vi "Archive Graduated Student.vi"(11 "BYU ID # In":string) -> ()   [LabVIEW 2019]
uses:
  Controls/Table Data Types/User Data Type.ctl
  Controls/Table Data Types/User Archive Data Type.ctl
  <vilib>/addons/database/Connection.llb/DB Tools Open Connec (String).vi
  <vilib>/addons/database/_DB Variant To Data/Database Variant To Data.xnode
  <vilib>/addons/database/NI_Database_API.lvlib
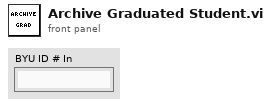
[diagram p1: front panel]
types:
  T1 = typedef "User Archive Data Type.ctl" = cluster{"BYU ID #":string, "First Name":string, "Last Name":string, "Phone Number":string, "Email":string, "Department":string, "Graduation Status":string, "Anticipated Graduation Year":string, "Credit Score":dbl, "Date Added":string, "Graduation Clearance Date":string, "Picture File Name":string, "Date Archived":string}
  T2 = typedef "User Data Type.ctl" = cluster{"BYU ID #":string, "First Name":string, "Last Name":string, "Phone Number":string, "Email":string, "Department":string, "Graduation Status":string, "Anticipated Graduation Year":string, "Credit Score":dbl, "Date Added":string, "Graduation Clearance Date":string, "Picture File Name":string, "User Comments":string}
  T3 = typedef "NI_Database_API.lvlib/Conn ObjectReference.ctl" = refnum<k1>
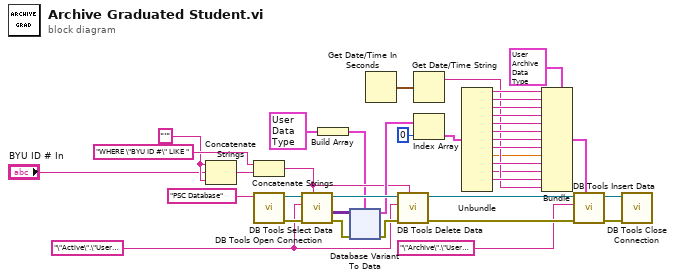
[diagram p0: block diagram]
diagram:
  w2 = "'" ("string")
  w16 = "\"Active\".\"Users\""
  n1 = Concatenate Strings(w2, "BYU ID # In", w2) -> (w3:string)
  n2 = Concatenate Strings("WHERE \"BYU ID #\" LIKE " ("string"), w3) -> (w17:string)
  n3 = call-poly <vilib>:"DB Tools Open Connection.vi"("connection information"="PSC Database") -> ("error out"=w37:errorcluster, "connection reference"=w38:T3)  [unwired: 7 in]
  n4 = call <vilib>:"DB Tools Select Data.vi"("condition"=w17, "error in (no error)"=w37, "table"=w16, "connection reference"=w38) -> ("error out"=w34:errorcluster, "data"=w35:variant[][], "connection reference out"=w36:T3)  [unwired: 2 in]
  n5 = Build Array(T2 {"BYU ID #"="", "First Name"="", "Last Name"="", "Phone Number"="", "Email"="", "Department"="", "Graduation Status"="", "Anticipated Graduation Year"="", "Credit Score"=0.0, "Date Added"="", "Graduation Clearance Date"="", "Picture File Name"="", "User Comments"=""} ("Array")) -> (w8:T2[])
  n6 = xnode "Database Variant To Data"("database variant"=w35, "error in (no error)"=w34, "type"=w8) -> ("data"=w32:T2[], "error out"=w33:errorcluster)
  n7 = Get Date/Time In Seconds() -> (seconds since 1Jan1904=w19:timestamp)
  n8 = call <vilib>:"DB Tools Delete Data.vi"("condition"=w17, "error in (no error)"=w33, "table"=w16, "connection reference"=w36) -> ("error out"=w13:errorcluster, "connection reference out"=w14:T3)  [unwired: 6 in]
  n9 = Get Date/Time String(seconds (now)=w19) -> (date string=w18:string)  [unwired: 2 in, 1 out]
  n10 = Index Array(array=w32, index=0) -> (element=w30:T2)
  n11 = Unbundle(w30) -> ("BYU ID #"=w29:string, "First Name"=w28:string, "Last Name"=w27:string, "Phone Number"=w26:string, "Email"=w25:string, "Department"=w24:string, "Graduation Status"=w23:string, "Anticipated Graduation Year"=w22:string, "Credit Score"=w6:dbl, "Date Added"=w21:string, "Graduation Clearance Date"=w5:string, "Picture File Name"=w20:string)  [unwired: 1 out]
  n12 = Bundle(cluster=T1 {"BYU ID #"="", "First Name"="", "Last Name"="", "Phone Number"="", "Email"="", "Department"="", "Graduation Status"="", "Anticipated Graduation Year"="", "Credit Score"=0.0, "Date Added"="", "Graduation Clearance Date"="", "Picture File Name"="", "Date Archived"=""} ("USER ARCHIVE DATA TYPE"), "BYU ID #"=w29, "First Name"=w28, "Last Name"=w27, "Phone Number"=w26, "Email"=w25, "Department"=w24, "Graduation Status"=w23, "Anticipated Graduation Year"=w22, "Credit Score"=w6, "Date Added"=w21, "Graduation Clearance Date"=w5, "Picture File Name"=w20, "Date Archived"=w18) -> (w15:T1)
  n13 = call <vilib>:"DB Tools Insert Data.vi"("data"=w15, "error in (no error)"=w13, "table"="\"Archive\".\"Users\"", "connection reference"=w14) -> ("error out"=w10:errorcluster, "connection reference out"=w11:T3)  [unwired: 6 in]
  n14 = call <vilib>:"DB Tools Close Connection.vi"("error in (no error)"=w10, "connection reference"=w11) -> ()  [unwired: 5 in, 1 out]
